vi "ACC_LabVIEW_LV_UnbundleData.vi"(1 "Acc_Data_In":T1[](array[typedef])) -> (15 "LV_double_array":dbl[](array[numeric]), 16 "LV_types":i32[](array[numeric]), 17 "Length":i32, 18 "Data-String":string)   [LabVIEW 2014, in "ACC_LabVIEW.lvlib"]
doc: "transforms the Acc data format to a double Array, a Type Array and a string"
uses:
  ACC_LabVIEW.lvlib
  ACC_LabVIEW_Container.ctl
  ACC_LabVIEW_DataTypes.ctl
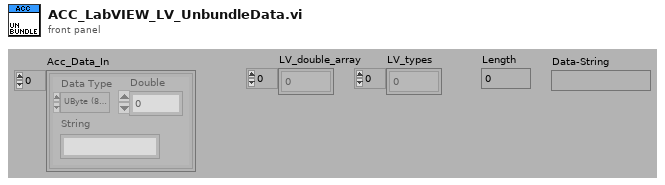
[diagram p1: front panel]
types:
  T1 = typedef "ACC_LabVIEW.lvlib/ACC_LabVIEW_Container.ctl" = cluster{"Data Type":T2, "String":string, "Double":dbl}
  T2 = typedef "ACC_LabVIEW.lvlib/ACC_LabVIEW_DataTypes.ctl" = enum16{"SByte (8Bit Int signed)", "UByte (8Bit int unsigned)", "SWord (16Bit Int signed)", "UWord (16Bit Int unsigned)", "SLong (32Bit Int signed)", "ULong (32Bit Int unsigned)", "Float32 (float)", "Float64 (double)", "String"}
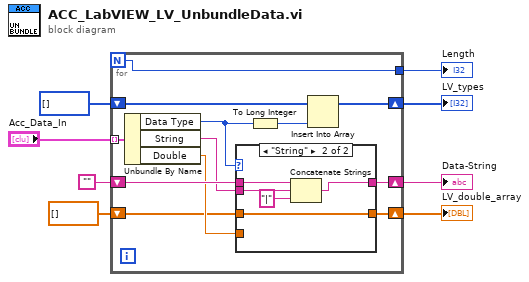
[diagram p0: block diagram]
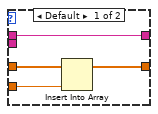
[diagram p2: hidden frame]
diagram:
  n1 = for {
    N -> [w9]
    shift-right: [w10] -> w7
    shift-left: dbl[] [] ("LV_para") -> [w11]
    shift-right: [w18] -> w6
    shift-left: i32[] [] ("LV_para_types") -> [w19]
    tunnel: "Acc_Data_In" -> [w20] mode=indexing
    shift-right: [w13] -> w8
    shift-left: "" -> [w15]
    tunnel: [w9] -> w1
    n2 = Unbundle By Name(w20) -> ("Data Type"=w16:T2, "String"=w14:string, "Double"=w12:dbl)
    n3 = case shown="\"String\"" w16 {
      tunnel: w15 -> [w24 w29]
      tunnel: w14 -> [_ w28]
      tunnel: [w24 w27] -> w13
      tunnel: w12 -> [w23 _]
      tunnel: w11 -> [w22 w25]
      tunnel: [w21 w25] -> w10
      frame Default {
        n4 = Insert Into Array(array=w22, new element=w23) -> (w21:dbl[])  [unwired: 1 in]
      }
      frame "String" {
        n5 = Concatenate Strings(w29, w28, "|") -> (w27:string)
      }
    }
    n6 = To Long Integer(number=w16) -> (32bit integer=w17:i32)
    n7 = Insert Into Array(array=w19, new element=w17) -> (w18:i32[])  [unwired: 1 in]
  }
  "Data-String" <- w8
  "LV_double_array" <- w7
  "Length" <- w1
  "LV_types" <- w6
